vi "output.vi"(8 "error in":errorcluster, 10 "data table in":T1, 11 "TDMS datalogger runtime in":refnum<class "TDMS datalogger runtime.lvclass">) -> (0 "error out":errorcluster, 2 "data table out":T1, 3 "TDMS datalogger runtime out":refnum<class "TDMS datalogger runtime.lvclass">)   [LabVIEW 2013, in "TDMS datalogger runtime.lvclass"]
doc: "Provides an interface for writing data to a module at runtime. While this interface performs no operations, a child should provide an override which may write to any open sessions, references, or interfaces."
uses:
  TDMS datalogger runtime.lvclass
  <vilib>/NI/Tag Bus/table/data table.ctl
  TDMS datalogger runtime.lvclass/TDMS datalogger runtime.ctl
  <vilib>/NI/Tag Bus/table/data table.lvlib
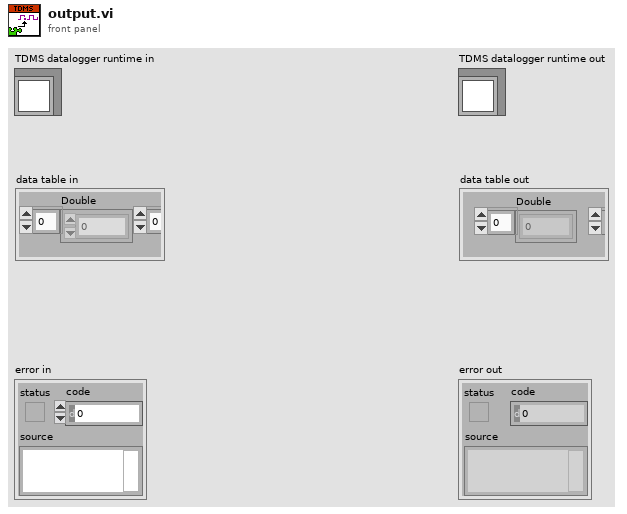
[diagram p1: front panel]
types:
  T1 = typedef "tag bus.lvlib/data table.lvlib/data table.ctl" = cluster{"Double":dbl[], "Single":sgl[], "I64":i64[], "I32":i32[], "I16":i16[], "I8":i8[], "U64":u64[], "U32":u32[], "U16":u16[], "U8":u8[], "Boolean":bool[], "String":string[], "Array of Double":cluster{"DBL Array":dbl[]}[], "Array of Single":cluster{"SGL Array":sgl[]}[], "Array of I64":cluster{"I64 Array":i64[]}[], "Array of I32":cluster{"I32 Array":i32[]}[], "Array of I16":cluster{"I16 Array":i16[]}[], "Array of I8":cluster{"I8 Array":i8[]}[], "Array of U64":cluster{"U64 Array":u64[]}[], "Array of U32":cluster{"U32 Array":u32[]}[], "Array of U16":cluster{"U16 Array":u16[]}[], "Array of U8":cluster{"U8 Array":u8[]}[], "Array of Boolean":cluster{"Boolean Array":bool[]}[], "Array of String":cluster{"String Array":string[]}[]}
  T2 = typedef "TDMS datalogger runtime.lvclass/sample queue.ctl" = cluster{"data to processor":refnum<queue>, "time to processor":refnum<queue>}
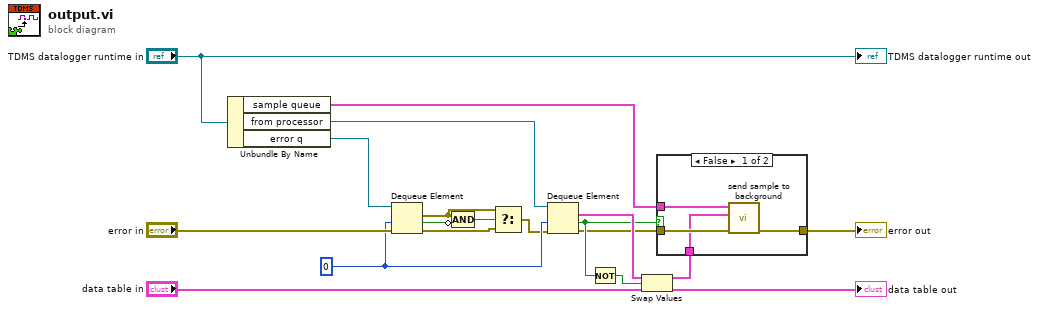
[diagram p0: block diagram]
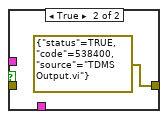
[diagram p2: hidden frame]
diagram:
  w6 = 0 ("timeout in ms (-1)")
  n1 = Unbundle By Name("TDMS datalogger runtime in") -> ("sample queue"=w17:T2, "from processor"=w16:refnum<queue>, "error q"=w15:refnum<queue>)
  n2 = Dequeue Element(queue=w15, timeout in ms (-1)=w6, error in (no error)="error in") -> (element=w3:errorcluster, timed out?=w5:bool, error out=w2:errorcluster)  [unwired: 1 out]
  n3 = Compound Arithmetic op=AND(w3, invert w5) -> (w4:bool)
  n4 = Select(t=w3, s=w4, f=w2) -> (s? t:f=w1:errorcluster)
  n5 = Dequeue Element(queue=w16, timeout in ms (-1)=w6, error in (no error)=w1) -> (element=w13:T1, timed out?=w10:bool, error out=w8:errorcluster)  [unwired: 1 out]
  n6 = Not(x=w10) -> (.not. x?=w11:bool)
  n7 = Swap Values(12:w13, 13:w11, 14:"data table in") -> (1:w12:T1, 3:→"data table out":T1)
  n8 = case shown="False" w10 {
    tunnel: w8 -> [w22 _]
    tunnel: w12 -> [w21 _]
    tunnel: w17 -> [w20 _]
    tunnel: [w23 errorcluster {"status"=TRUE, "code"=538400, "source"="TDMS Output.vi"} ("error out")] -> w7
    frame False {
      n9 = call "send sample to background.vi"("error in"=w22, "data table"=w21, "sample queue"=w20) -> ("error out"=w23:errorcluster)  [unwired: 8 in]
    }
    frame True {
    }
  }
  "error out" <- w7
  "TDMS datalogger runtime out" <- "TDMS datalogger runtime in"
